vi "kvCanObjBufFree.vi"(2 "error in (no error)":errorcluster, 3 "Object Handle":i32, 4 "Channel Handle (input only)":i32) -> (0 "error out":errorcluster, 1 "Channel Handle (output only)":i32)   [LabVIEW 2022 SP3]
doc: "Releases the specified object handle associated with the CAN circuit back to the object pool."
uses:
  canlib32.dll
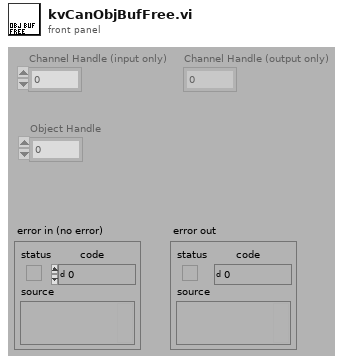
[diagram p1: front panel]
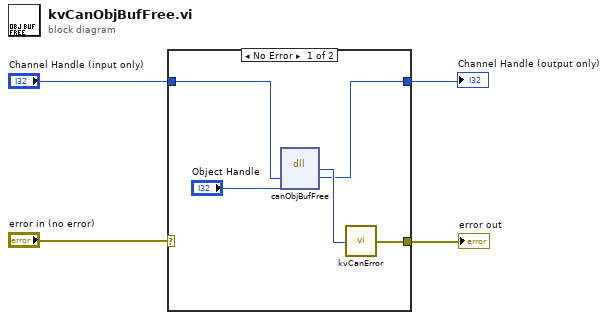
[diagram p0: block diagram]
diagram:
  n1 = case shown="No Error" "error in (no error)" {
    selector: "error in (no error)" -> [_ w11]
    tunnel: [w9 w11] -> w3
    tunnel: "Channel Handle (input only)" -> [w7 w10]
    tunnel: [w5 w10] -> w1
    frame No Error {
      n2 = dll-call lib="canlib32.dll" fn="canObjBufFree"("channelHandle"=w7, "objectHandle"="Object Handle") -> (w6:i32, "channelHandle"=w5:i32)  [unwired: 4 in, 2 out]
      n3 = call "kvCanError.vi"("error code"=w6) -> ("error out"=w9:errorcluster)
    }
    frame Error {
    }
  }
  "Channel Handle (output only)" <- w1
  "error out" <- w3
